vi "ArmConveyor Controller.vi"(8 "error in":errorcluster) -> ()   [LabVIEW 2019]
doc: "This VI executes continuously carrying out the current operation and responding to updates or new operations. It will often contain the timing or control code that is difficult to place directly in TeleOp. This VI generally opens all sensors and motors and isolates the rest of the robot code from knowing how the operations are carried out."
uses:
  <vilib>/Rock Robotics/WPI/Framework/Completion Status.ctl
  ArmConveyor Setpoints.ctl
  ArmConveyor Operations.ctl
  <vilib>/Rock Robotics/WPI/SafetyOutput/WPI_SafetyOutputConfigMenu.ctl
  <vilib>/Rock Robotics/Network Tables/NT Write Boolean.vi
panel:
  in  "Interactive Values":T1
  out "Current\nCmd":string
  in  "Buttons":cluster{"Execute Cmd":bool, "Abort Cmd":bool}
  out "Command Timing":cluster{"Start Time (ms)":u32, "Iterations":i32}
  out "Status":T3
  # "Tip: It may be helpful to observe inputs and sensor values.\nYou may also want to display tuning or debugging controls."
  # "Interactive Command: You may fill in the settings for a command\nand schedule it with the Execute button. You can observe and abort\nany command while fine tuning the code for the controller."
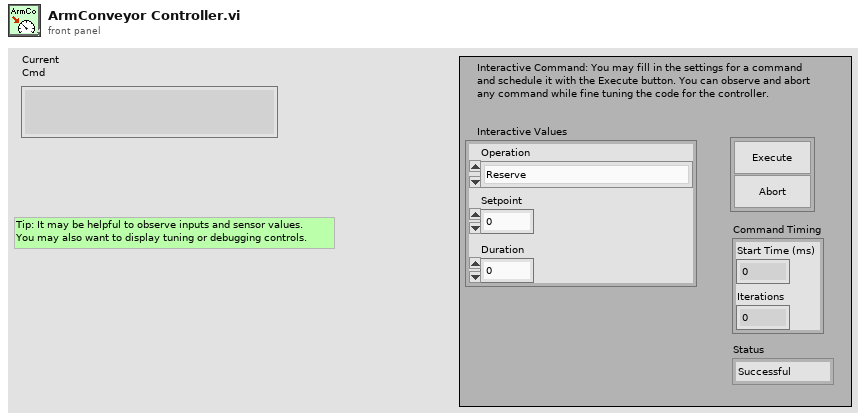
[diagram p1: front panel]
types:
  T1 = typedef "ArmConveyor Setpoints.ctl" = cluster{"Operation":T2, "Setpoint":dbl, "Duration":dbl}
  T2 = typedef "ArmConveyor Operations.ctl" = enum16{"Reserve", "Read Current", "Immediate", "Arm Conveyor Duration"}
  T3 = typedef "Completion Status.ctl" = enum16{"Successful", "Aborted", "Incomplete"}
  T4 = typedef "WPI_SafetyOutputConfigMenu.ctl" = enum16{"Enable", "Disable"}
  T5 = typedef "WPI_MotorControlDeviceRef.ctl" = cluster{"DeviceStatus":errorcluster, "Type":T6, "PWM":cluster{"PWM Channel":T7, "DeadBand":T8}, "CAN":cluster{"Device Number":u8, "SetOutput VI Ref":variant, "GetOutput VI Ref":variant, "Enable VI Ref":variant, "Disable VI Ref":variant, "Data":variant}, "Invert":bool, "DIO PWM":cluster{"PWM \"Enable\" Channel":T7, "DIOChannel":T9, "PWM Rate":dbl}}
  T6 = typedef "WPI_MotorControlType.ctl" = enum16{"PWM", "CAN", "DIO PWM"}
  T7 = typedef "FPGA_DIOPWMChannel.ctl" = enum8{"PWM 0", "PWM 1", "PWM 2", "PWM 3", "PWM 4", "PWM 5", "PWM 6", "PWM 7", "PWM 8", "PWM 9", "PWM MXP 0", "PWM MXP 1", "PWM MXP 2", "PWM MXP 3", "PWM MXP 4", "PWM MXP 5", "PWM MXP 6", "PWM MXP 7", "PWM MXP 8", "PWM MXP 9", "Invalid"}
  T8 = typedef "WPI_PWMDeadband.ctl" = cluster{"Name":string, "maxPositivePwm":i32, "minPositivePwm":i32, "centerPwm":i32, "maxNegativePwm":i32, "minNegativePwm":i32, "angularRange":u16}
  T9 = typedef "FPGA_DIOChannel.ctl" = enum8{"DIO 0", "DIO 1", "DIO 2", "DIO 3", "DIO 4", "DIO 5", "DIO 6", "DIO 7", "DIO 8", "DIO 9", "DIO MXP 0", "DIO MXP 1", "DIO MXP 2", "DIO MXP 3", "DIO MXP 4", "DIO MXP 5", "DIO MXP 6", "DIO MXP 7", "DIO MXP 8", "DIO MXP 9", "DIO MXP 10", "DIO MXP 11", "DIO MXP 12", "DIO MXP 13", "DIO MXP 14", "DIO MXP 15", "SPI Port CS1", "SPI Port CS2", "SPI Port CS3", "SPI Port MISO", "SPI Port MOSI", "Invalid"}
  T10 = typedef "Command Status Info.ctl" = cluster{"Name":string, "Status":T3, "notifier out":T11}
  T11 = typedef "Completion Notifier.ctl" = refnum<notifier>
  T12 = cluster{"Current Command":T1, "Command Timing":cluster{"Start Time (ms)":u32, "Iterations":i32}, "Command Arguments":cluster{"Command Info":T10, "Description":string, "Default Command":T1, "queue out":refnum<queue>, "Subsystem Name":string}}
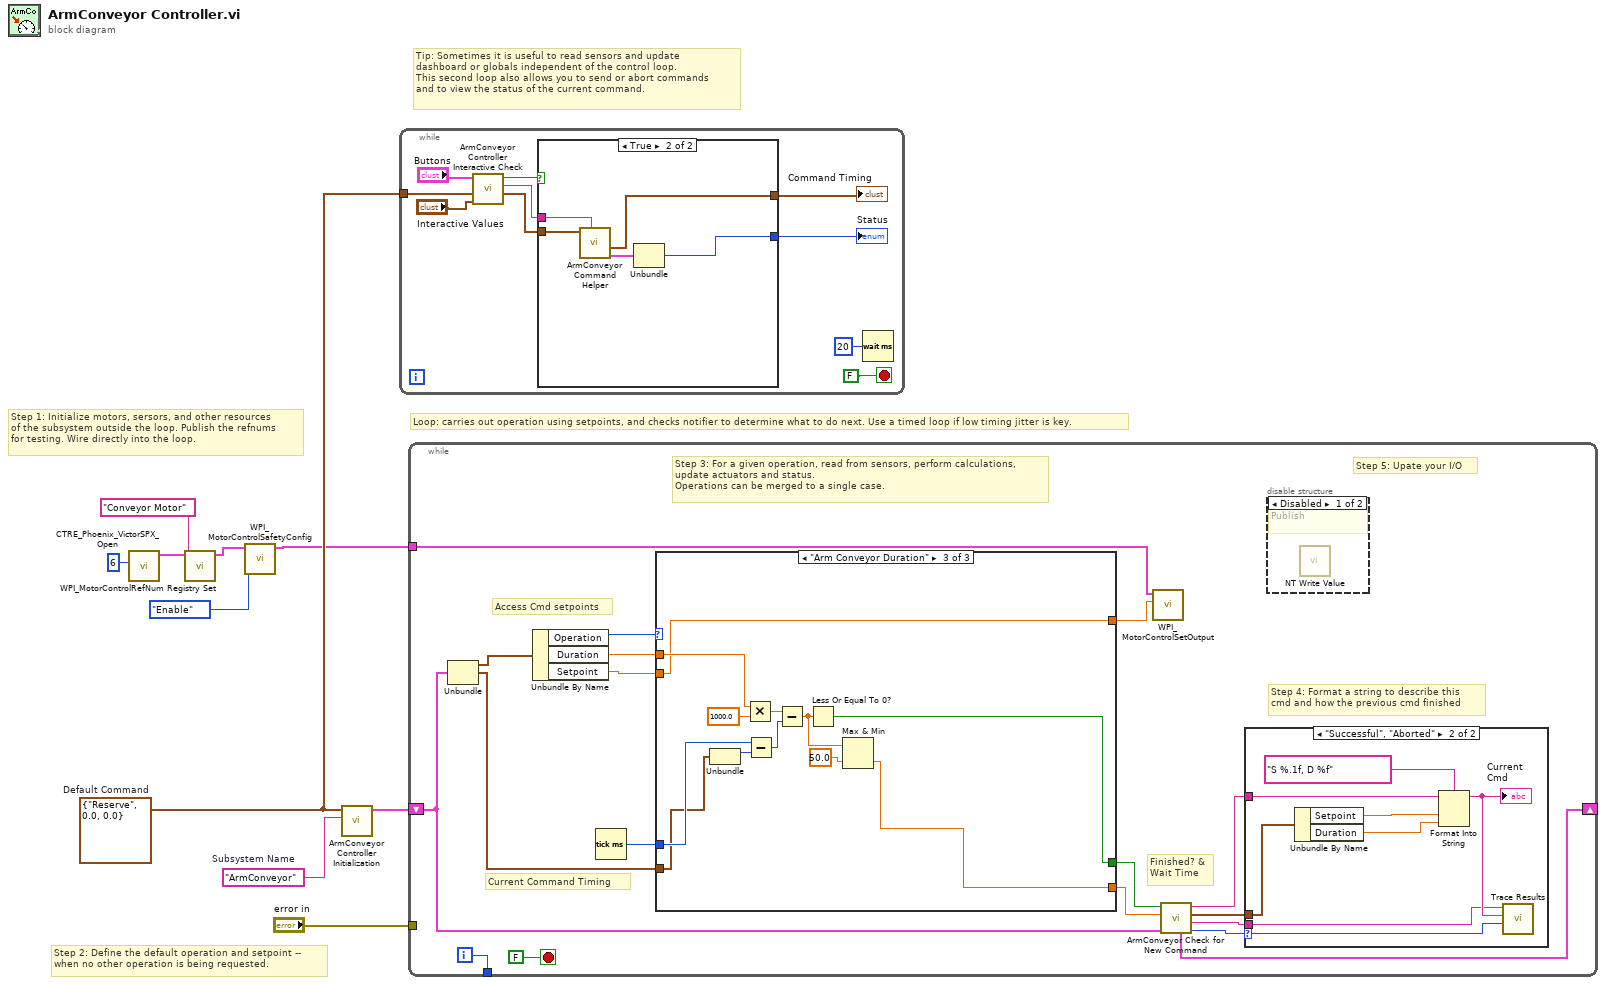
[diagram p0: block diagram]
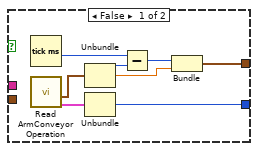
[diagram p2: hidden frame]
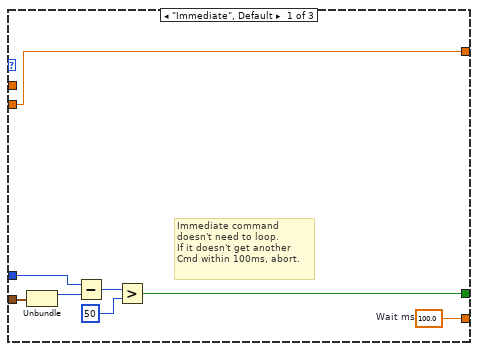
[diagram p5: hidden frame]
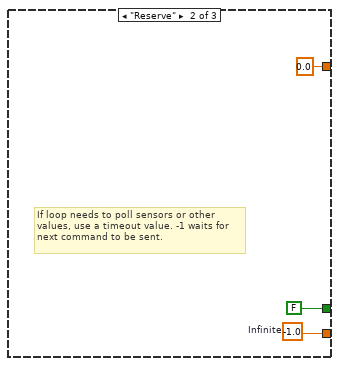
[diagram p6: hidden frame]
diagram:
  w7 = T1 {"Operation"=enum."Reserve", "Setpoint"=0.0, "Duration"=0.0}  # Default Command
  w8 = "ArmConveyor"  # Subsystem Name
  # "Tip: Sometimes it is useful to read sensors and update\ndashboard or globals independent of the control loop.\nThis second loop also allows you to send or abort commands\nand to view the status of the current command."
  # "Step 2: Define the default operation and setpoint --\nwhen no other operation is being requested."
  # "Step 1: Initialize motors, sersors, and other resources\nof the subsystem outside the loop. Publish the refnums\nfor testing. Wire directly into the loop."
  # "Loop: carries out operation using setpoints, and checks notifier to determine what to do next. Use a timed loop if low timing jitter is key."
  n1 = call <vilib>:"CTRE_Phoenix_VictorSPX_Open.vi"("Device Number"=u8 6) -> ("CAN Talon SRX Ref"=w5:T5)  [unwired: 9 in, 1 out]
  n2 = call <vilib>:"WPI_MotorControlRefNum Registry Set.vi"("refnum name"="Conveyor Motor", "MotorControlDevRef"=w5) -> ("MotorControlDevRef"=w3:T5)  [unwired: 8 in, 1 out]
  n3 = call <vilib>:"WPI_MotorControlSafetyConfig.vi"("mode"=WPI_SafetyOutputConfigMenu."Enable", "MotorControlDevRef"=w3) -> ("MotorControlDevRef"=w1:T5)  [unwired: 8 in, 1 out]
  n4 = call "ArmConveyor Controller Initialization.vi"("Subsystem Name"=w8, "Default Command"=w7) -> ("Current Command"=w9:T12)  [unwired: 9 in]
  n5 = while {
    tunnel: w7 -> [w17]
    stop <- FALSE stop-if-true
    n6 = call "ArmConveyor Controller Interactive Check.vi"("Interactive Command in"="Interactive Values", "Default Command"=w17, "Buttons"="Buttons") -> ("Interactive Command out"=w14:T1, "Trace String"=w15:string, "Schedule"=w16:bool)  [unwired: 6 in]
    n7 = case shown="True" w16 {
      tunnel: [w28 w33] -> w13
      tunnel: w14 -> [_ w31]
      tunnel: [w24 w29] -> w12
      tunnel: w15 -> [_ w32]
      frame False {
        n8 = Tick Count (ms)() -> (millisecond timer value=w23:u32)
        n9 = call "Read ArmConveyor Operation.vi"() -> ("Command Info"=w21:T10, "SubSystem Data"=w22:T1)  [unwired: 9 in, 1 out]
        n10 = Unbundle(w22) -> ("Operation"=w27:T2, "Setpoint"=w25:dbl)  [unwired: 1 out]
        n11 = Unbundle(w21) -> ("Status"=w28:T3)  [unwired: 2 out]
        n12 = Subtract(x=w23, y=w27) -> (x-y=w26:u32)
        n13 = Bundle(w26, "Setpoint"=w25) -> (w24:cluster{u32, "Setpoint":dbl})  [unwired: 1 in]
      }
      frame True {
        n14 = call "ArmConveyor Command Helper.vi"("Description"=w32, "SubSystem Data"=w31) -> ("Command Info Out"=w30:T10, "Command Timing"=w29:cluster{"Start Time (ms)":u32, "Iterations":i32})  [unwired: 7 in, 1 out]
        n15 = Unbundle(w30) -> ("Status"=w33:T3)  [unwired: 2 out]
      }
    }
    "Status" <- w13
    "Command Timing" <- w12
    n16 = Wait (ms)(milliseconds to wait=u32 20) -> ()  [unwired: 1 out]
  }
  n17 = while {
    shift-right: [w43] -> _
    shift-left: w9 -> [w36]
    tunnel: [w50] -> _
    tunnel: "error in" -> [_]
    tunnel: w1 -> [w35]
    i -> [w50]
    stop <- FALSE stop-if-true
    # "Step 5: Upate your I/O"
    # "Step 4: Format a string to describe this\ncmd and how the previous cmd finished"
    # "Current Command Timing"
    # "Access Cmd setpoints"
    # "Finished? &\nWait Time"
    # "Step 3: For a given operation, read from sensors, perform calculations,\nupdate actuators and status.\nOperations can be merged to a single case."
    n18 = Unbundle(w36) -> ("Current Command"=w49:T1, "Command Timing"=w45:cluster{"Start Time (ms)":u32, "Iterations":i32})  [unwired: 1 out]
    n19 = Unbundle By Name(w49) -> ("Operation"=w48:T2, "Duration"=w47:dbl, "Setpoint"=w44:dbl)
    n20 = Tick Count (ms)() -> (millisecond timer value=w46:u32)
    n21 = case shown="\"Arm Conveyor Duration\"" w48 {
      tunnel: [w67 w70 w71] -> w41
      tunnel: [w61 FALSE ("ignore previous (F)") w72] -> w42
      tunnel: w45 -> [w63 _ w75]
      tunnel: w47 -> [_ _ w74]
      tunnel: w46 -> [w62 _ w76]
      tunnel: w44 -> [w60 _ w73]
      tunnel: [w60 0.0 ("Setpoint") w73] -> w34
      frame "Immediate", Default {
        w67 = 100.0  # Wait ms
        # "Immediate command\ndoesn't need to loop.\nIf it doesn't get another\nCmd within 100ms, abort."
        n22 = Unbundle(w63) -> ("Start Time (ms)"=w66:u32)  [unwired: 1 out]
        n23 = Subtract(x=w62, y=w66) -> (x-y=w65:u32)
        n24 = Greater?(x=w65, y=u8 50 ("Left Motor")) -> (0:w61:bool)
      }
      frame "Reserve" {
        w70 = -1.0  # Infinite
        # "If loop needs to poll sensors or other\nvalues, use a timeout value. -1 waits for\nnext command to be sent."
      }
      frame "Arm Conveyor Duration" {
        n25 = Unbundle(w75) -> ("Start Time (ms)"=w79:u32)  [unwired: 1 out]
        n26 = Multiply(x=w74, y=1000.0) -> (x*y=w81:dbl)
        n27 = Subtract(x=w76, y=w79) -> (x-y=w82:u32)
        n28 = Subtract(x=w81, y=w82) -> (x-y=w78:dbl)
        n29 = Less Or Equal To 0?(x=w78) -> (x <= 0?=w72:bool)
        n30 = Max & Min(x=w78, y=50.0) -> (min(x,y)=w71:dbl)  [unwired: 1 out]
      }
    }
    n31 = call <vilib>:"WPI_MotorControlSetOutput.vi"("Output"=w34, "MotorControlDevRef"=w35) -> ()  [unwired: 7 in, 3 out]
    n32 = call "ArmConveyor Check for New Command.vi"("Current Command"=w36, "Wait time (ms)"=w41, "Finished?"=w42) -> ("Completion"=w37:T3, "Subsystem Name"=w38:string, "Current Command"=w39:T1, "Initial Trace String"=w40:string, "NextCommand"=w43:T12)  [unwired: 4 in]
    n33 = case shown="\"Successful\", \"Aborted\"" w37 {
      selector: w37 -> [_ w59]
      tunnel: w40 -> [_ w55]
      tunnel: w39 -> [_ w56]
      tunnel: w38 -> [_ w52]
      frame "Incomplete", Default {
        # "Continuing current command"
      }
      frame "Successful", "Aborted" {
        # "Report and setup for next command"
        n34 = Unbundle By Name(w56) -> ("Setpoint"=w58:dbl, "Duration"=w53:dbl)
        n35 = Format Into String(format string="S %.1f, D %f", initial string=w55, w58, w53) -> (resulting string=w54:string)  [unwired: 1 in, 1 out]
        "Current\nCmd" <- w54
        n36 = call <vilib>:"Trace Results.vi"("Status of previous command"=w59, "Description"=w54, "Subsystem"=w52) -> ()  [unwired: 9 in]
      }
    }
    n37 = disable-structure shown="Disabled" {
      frame Disabled {
        # "Publish"
        n38 = call-poly <vilib>:"NT Write Value.vi"() -> ()  [unwired: 11 in, 1 out]
      }
      frame Enabled {
      }
    }
  }
